vi "Log Debug(by Ref).vi"(10 "error in (no error)":errorcluster, 11 "Message":string) -> (2 "error out":errorcluster)   [LabVIEW 2017, in "Error Log.lvlib" / "Logger.lvclass"]
doc: "Logs an event with level Debug to the referenced ``*Logger``."
uses:
  Logger.lvclass
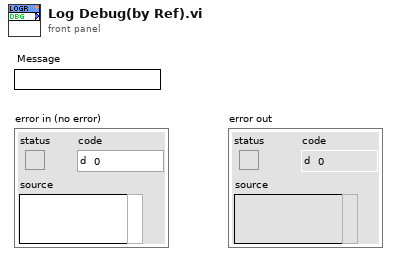
[diagram p1: front panel]
types:
  T1 = enum16{"DEBUG", "INFO", "WARNING", "ERROR", "CRITICAL"}
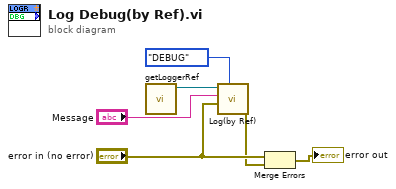
[diagram p0: block diagram]
diagram:
  n1 = call "getLoggerRef.vi"() -> ("Logger Ref"=w4:refnum<data-value>)  [unwired: 10 in, 1 out]
  n2 = call "Log(by Ref).vi"("Level"=T1."DEBUG", "error"="error in (no error)", "Message"="Message", "Logger Ref in"=w4) -> ("error out"=w1:errorcluster)  [unwired: 6 in, 1 out]
  n3 = Merge Errors("error in (no error)", w1) -> (→"error out":errorcluster)
